vi "05_Dialog.vi"() -> ()   [LabVIEW 2020]
uses:
  <vilib>/MGI/Panel Manager/Panel/Panel.lvlib
  <vilib>/MGI/Panel Manager/Panel/Window Position/Reference Position/Horizontal Alignment.ctl
  <vilib>/MGI/Panel Manager/Panel/Window Position/Reference Position/Reference Position.lvclass
  <vilib>/MGI/Panel Manager/Panel/Window Position/Reference Position/Vertical Alignment.ctl
  <vilib>/MGI/Panel Manager/Panel/Window Position/Reference Position/Alignment.ctl
  <vilib>/MGI/Panel Manager/Panel/Panel/Window/Window.lvclass
  <vilib>/MGI/Panel Manager/Panel/Panel/Panel.lvclass
  <vilib>/MGI/Panel Manager/Panel/Window Position/Reference Position/Ref Display/Ref Display.vi
  <vilib>/MGI/Panel Manager/Panel/Window Position/Reference Position/Ref Display/Ref Display.lvclass
  <vilib>/MGI/Panel Manager/Panel/Panel/Window/Window.vi
  C:/Program Files (x86)/National Instruments/LabVIEW 2023/vi.lib/MGI/Panel Manager/Panel/Window Position/Reference Position/Reference Position.lvclass
  C:/Program Files (x86)/National Instruments/LabVIEW 2023/vi.lib/MGI/Panel Manager/Panel/Window Position/Window Position.lvclass
  C:/Program Files (x86)/National Instruments/LabVIEW 2023/vi.lib/MGI/Panel Manager/Panel/Window Position/Reference Position/Ref Display/Ref Display.lvclass
  C:/Program Files (x86)/National Instruments/LabVIEW 2023/vi.lib/MGI/Panel Manager/Panel/Panel/Panel.lvclass
panel:
  in  "Open Dialog\nWindow":bool
  out "Dialog Result OK?":bool
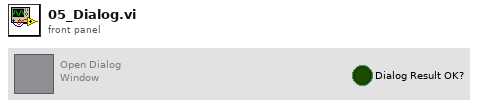
[diagram p1: front panel]
types:
  T1 = typedef "Panel.lvlib/Reference Position.lvclass/Alignment.ctl" = cluster{"Horizontal":T2, "Vertical":T3}
  T2 = typedef "Panel.lvlib/Reference Position.lvclass/Horizontal Alignment.ctl" = enum16{"Left", "Center", "Right"}
  T3 = typedef "Panel.lvlib/Reference Position.lvclass/Vertical Alignment.ctl" = enum16{"Top", "Center", "Bottom"}
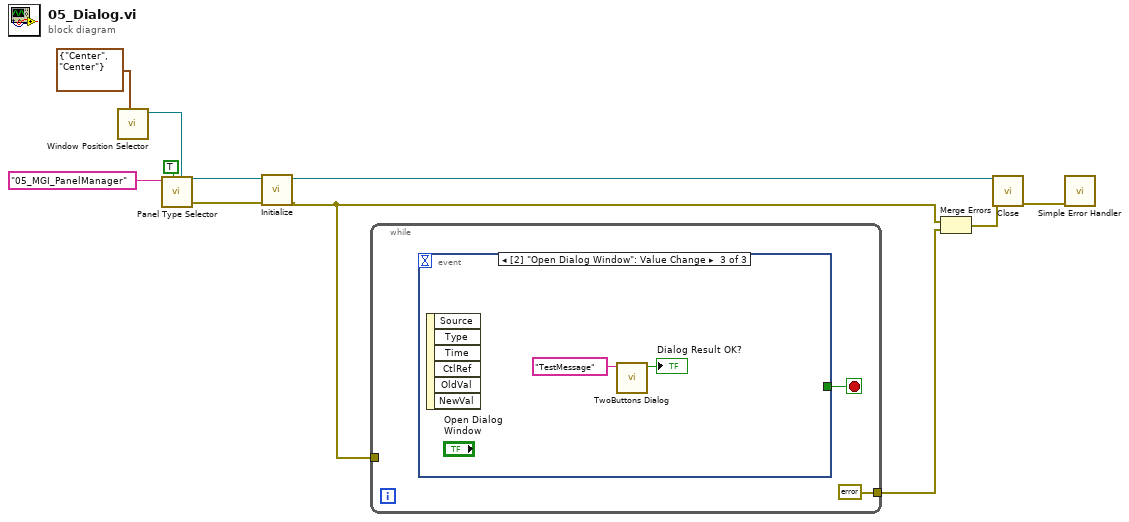
[diagram p0: block diagram]
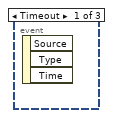
[diagram p2: hidden frame]
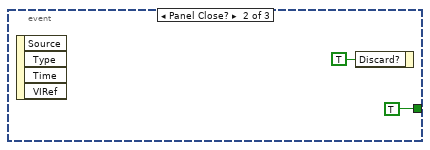
[diagram p3: hidden frame]
diagram:
  n1 = call-poly <vilib>:"Window Position Selector.vi"("Alignment"=T1 {"Horizontal"=enum."Center", "Vertical"=enum."Center"}) -> ("Ref Display out"=w8:refnum<class "Ref Display.lvclass">)  [unwired: 9 in, 1 out]
  n2 = call-poly <vilib>:"Panel Type Selector.vi"("Window Position"=w8, "Autoshow? (T)"=TRUE, "Default Title"="05_MGI_PanelManager") -> ("error out"=w3:errorcluster, "Window out"=w4:refnum<class "Window.lvclass">)  [unwired: 7 in]
  n3 = call <vilib>:"Initialize.vi"("error in (no error)"=w3, "Panel In"=w4) -> ("error out"=w2:errorcluster, "Panel Out"=w1:refnum<class "Window.lvclass">)  [unwired: 7 in, 1 out]
  n4 = while {
    tunnel: [errorcluster {"status"=FALSE, "code"=0, "source"=""} ("error constant")] -> w9
    tunnel: w2 -> [_]
    stop <- w13 stop-if-true
    n5 = event shown="[2] \"Open Dialog Window\": Value Change" {
      selector: _ -> [_ _ _]
      dyn-events: _ -> [_ _ _]
      timeout: _ -> [_ _ _]
      tunnel: [_ TRUE _] -> w13
      event Timeout {
        n6 = event-data() -> ()  [unwired: 1 in, 3 out]
      }
      event Panel Close? {
        n7 = event-data() -> ()  [unwired: 1 in, 4 out]
        n8 = event-data("Discard?"=TRUE) -> ()  [unwired: 1 in, 1 out]
      }
      event "Open Dialog\nWindow": Value Change {
        n9 = event-data() -> ()  [unwired: 1 in, 6 out]
        n10 = call "TwoButtons Dialog.vi"("Message"="TestMessage") -> ("OK?"=→"Dialog Result OK?":bool)  [unwired: 9 in, 1 out]
      }
    }
  }
  n11 = Merge Errors(w2, w9) -> (w10:errorcluster)
  n12 = call-dynamic "Close.vi"("error in (no error)"=w10, "UI Element in"=w1) -> ("error out"=w5:errorcluster)  [unwired: 9 in]
  n13 = call <vilib>:"Simple Error Handler.vi"("error in (no error)"=w5) -> ()  [unwired: 4 in, 5 out]
